vi "LocalQuadraticSumArrays.vi"(10 "size(s)":i16[](array[numeric]), 11 "Image Pixels (U8)":u8[][](array[numeric])) -> (3 "localsum":dbl[][](array[numeric]))   [LabVIEW 2014]
uses:
  <vilib>/imath/engines/lvmath2/RunTimeEngine/BuiltInFunctions/padarray/NIMS_padarray(GM).vi
  <instcachedir>/0/NIMS_padarray(GM)_7770B95E7B0443CF931C9D53726FB328.lvgen/NIMS_padarray(GM)_7770B95E7B0443CF931C9D53726FB328_003.vi
  <vilib>/imathl/engines/lvmath/Functions/Error Handling/Create Error.vi
  <vilib>/imath/engines/lvmath2/RunTimeEngine/BuiltInFunctions/accumsums/NIMS_accumsums(GM,Sca).vi
  <instcachedir>/0/NIMS_accumsums(GM,Sca)_61C6E63B19E747FC8144E869C786D277.lvgen/NIMS_accumsums(GM,Sca)_61C6E63B19E747FC8144E869C786D277_000.vi
  <vilib>/imath/engines/lvmath2/RunTimeEngine/IndexRead/NIMS V(S).vi
  <instcachedir>/0/NIMS V(S)_0488751826AF41519A22953C041130DC.lvgen/NIMS V(S)_0488751826AF41519A22953C041130DC_003.vi
  <vilib>/imath/engines/lvmath2/RunTimeEngine/IndexRead/NIMS M(R2,$).vi
  <instcachedir>/0/NIMS M(R2,$)_AD8DC2FC79024024B2717E13B4A0EB4B.lvgen/NIMS M(R2,$)_AD8DC2FC79024024B2717E13B4A0EB4B_000.vi
  <vilib>/imath/engines/lvmath2/RunTimeEngine/ArithmeticOperatorToken/NIMS_ArithmeticOperator_minus.vi
  <instcachedir>/0/NIMS_ArithmeticOperator_minus_39C0593E74DA4138ACA2AB742906488D.lvgen/NIMS_ArithmeticOperator_minus_39C0593E74DA4138ACA2AB742906488D_002.vi
  <vilib>/imath/engines/lvmath2/RunTimeEngine/ErrorHandling/NIMS_Create Error From Enums.vi
  <vilib>/imath/engines/lvmath2/RunTimeEngine/IndexRead/NIMS M($,R2).vi
  <instcachedir>/0/NIMS M($,R2)_D9380E19261A4ADFB2D364AF6959C6EF.lvgen/NIMS M($,R2)_D9380E19261A4ADFB2D364AF6959C6EF_001.vi
  <vilib>/imath/engines/lvmath2/RunTimeEngine/NodeEndStatement/NIMS_NodeEndStatement_Output.vi
  <instcachedir>/0/NIMS_NodeEndStatement_Output_53EC0D466D134D7ABD903AC30B43404B.lvgen/NIMS_NodeEndStatement_Output_53EC0D466D134D7ABD903AC30B43404B_002.vi
  <vilib>/imath/engines/lvmath2/RunTimeEngine/ErrorHandling/NIMS_Finalize Error.vi
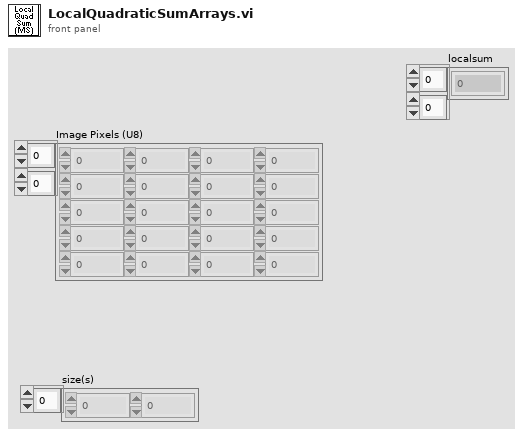
[diagram p1: front panel]
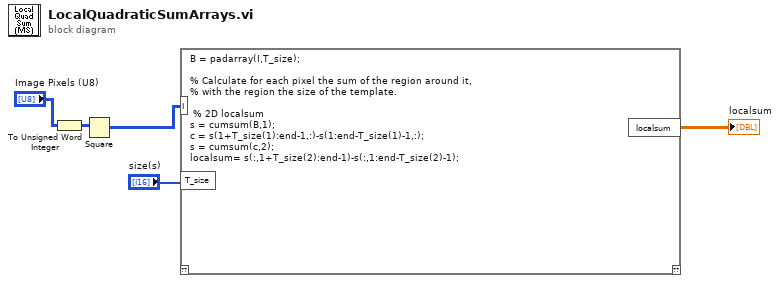
[diagram p0: block diagram]
diagram:
  n1 = To Unsigned Word Integer(number="Image Pixels (U8)") -> (unsigned 16bit integer=w3:u16[][])
  n2 = Square(x=w3) -> (x^2=w2:u16[][])
  n3 = mathscript code="B = padarray(I,T_size);\n\n% Calculate for each pixel the sum of the region around it,\n% with the region the size of the template.\n\n % 2D localsum\ns = cumsum(B,1);\nc = s(1+T_size(1):end-1,:)-s(1:end-T_size(1)-1,:);\ns = cumsum(c,2);\nlocalsum= s(:,1+T_size(2):end-1)-s(:,1:end-T_size(2)-1);"("I"=w2, "T_size"="size(s)") -> ("localsum"=→"localsum":dbl[][])  [unwired: 1 in, 1 out]
